vi "dfd_nMAC_CircSubN.vi"(1 "len":fxp<+,16,16>, 2 "idxIn":fxp<+,16,16>, 4 "step":fxp<+,16,16>) -> (6 "wrap?":bool, 7 "idxOut":fxp<+,16,16>)   [LabVIEW 2017]
uses:
  <vilib>/rvi/FXPMathLib/basic elements/FxpAddSub/XNode/nifxpmath_AddSub.xnode
  <vilib>/rvi/FXPMathLib/sim/FxpSim.dll
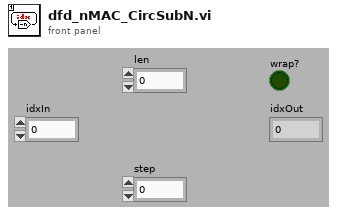
[diagram p1: front panel]
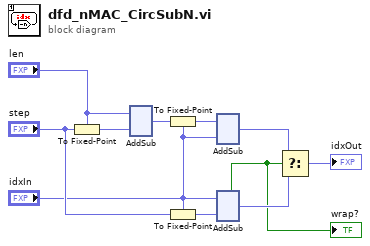
[diagram p0: block diagram]
diagram:
  n1 = To Fixed-Point(fixed-point type="len", number="step") -> (fixed-point=w5:fxp<+,16,16>)
  n2 = xnode "AddSub"("x"="len", "y"=w5) -> ("s"=w6:fxp<+,16,16>)  [unwired: 1 out]
  n3 = To Fixed-Point(fixed-point type="idxIn", number=w6) -> (fixed-point=w3:fxp<+,16,16>)
  n4 = To Fixed-Point(fixed-point type="idxIn", number="step") -> (fixed-point=w2:fxp<+,16,16>)
  n5 = xnode "AddSub"("x"=w3, "y"="idxIn") -> ("s"=w11:fxp<+,16,16>)  [unwired: 1 out]
  n6 = xnode "AddSub"("x"="idxIn", "y"=w2) -> ("s"=w10:fxp<+,16,16>, "borrow-out"=w9:bool)
  "wrap?" <- w9
  n7 = Select(t=w11, s=w9, f=w10) -> (s? t:f=→"idxOut":fxp<+,16,16>)
